vi "main_representacion.vi"(10 "Datos Leídos TyP":string[](array[string]), 11 "Datos Leídos Luz":string[](array[string])) -> ()   [LabVIEW 2021]
uses:
  Global 1.vi
panel:
  in  "Boolean 2":bool
  in  "Tab Control":T1(tab)
  out "Curvas luz y temperatura":cluster{"Ramp Pattern":dbl[], dbl[]}[](graph)
  in  "Load":bool
  in  "Export":bool
  in  "Curva de Luz":path
  in  "Curva de Temperatura":path
  in  "Ruta Luz":path
  in  "Ruta Temperatura":path
  in  "Integrate":bool
  in  "X1 (s)":dbl
  in  "X2 (s)":dbl
  out "Resultado":dbl
  in  "Load 2":bool
  in  "Load 3":bool
  out "Curvas  Luz":cluster{"Ramp Pattern":dbl[], u32[]}[](graph)
  in  "Luz 4":path
  in  "Luz 3":path
  in  "Luz 2":path
  in  "Luz 1":path
  in  "Temperatura 4":path
  in  "Temperatura 3":path
  in  "Temperatura 2":path
  in  "Temperatura 1":path
  out "Curvas Temperatura":cluster{"Ramp Pattern":dbl[], u32[]}[](graph)
  # "Glow Curves\nAnalysis"
  # "Área de integración"
  # "Curvas de Temperatura"
  # "Curvas de Luz"
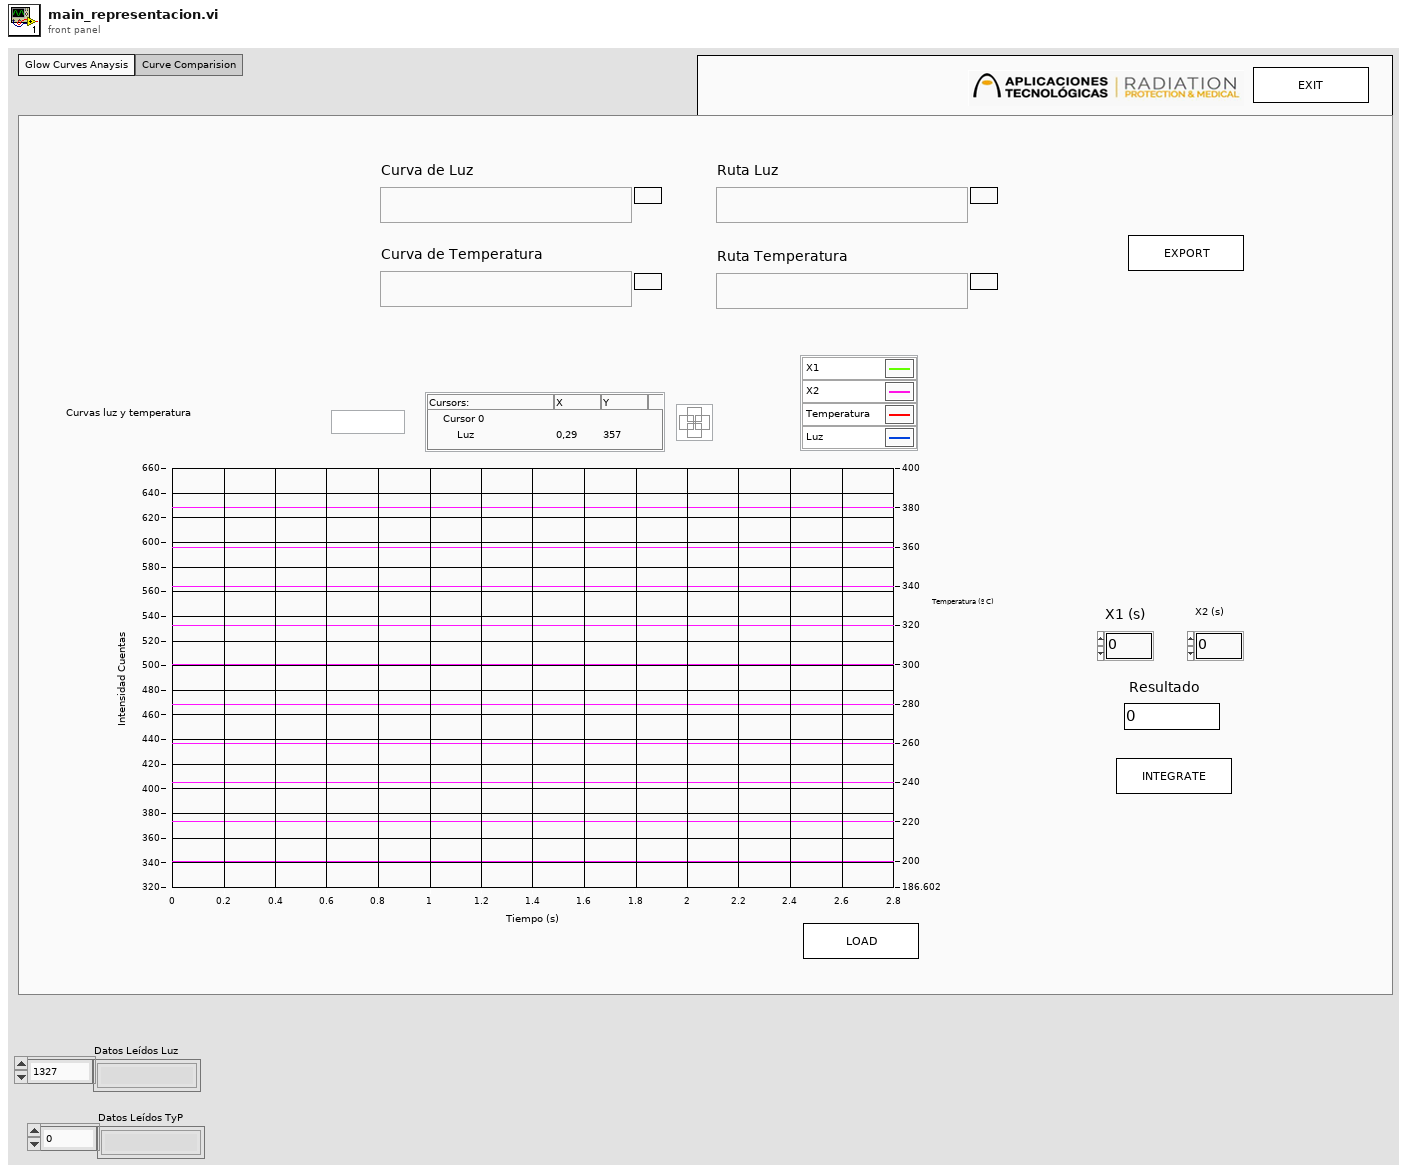
[diagram p1: front panel]
types:
  T1 = enum32{"Glow Curves Anaysis", "Curve Comparision"}
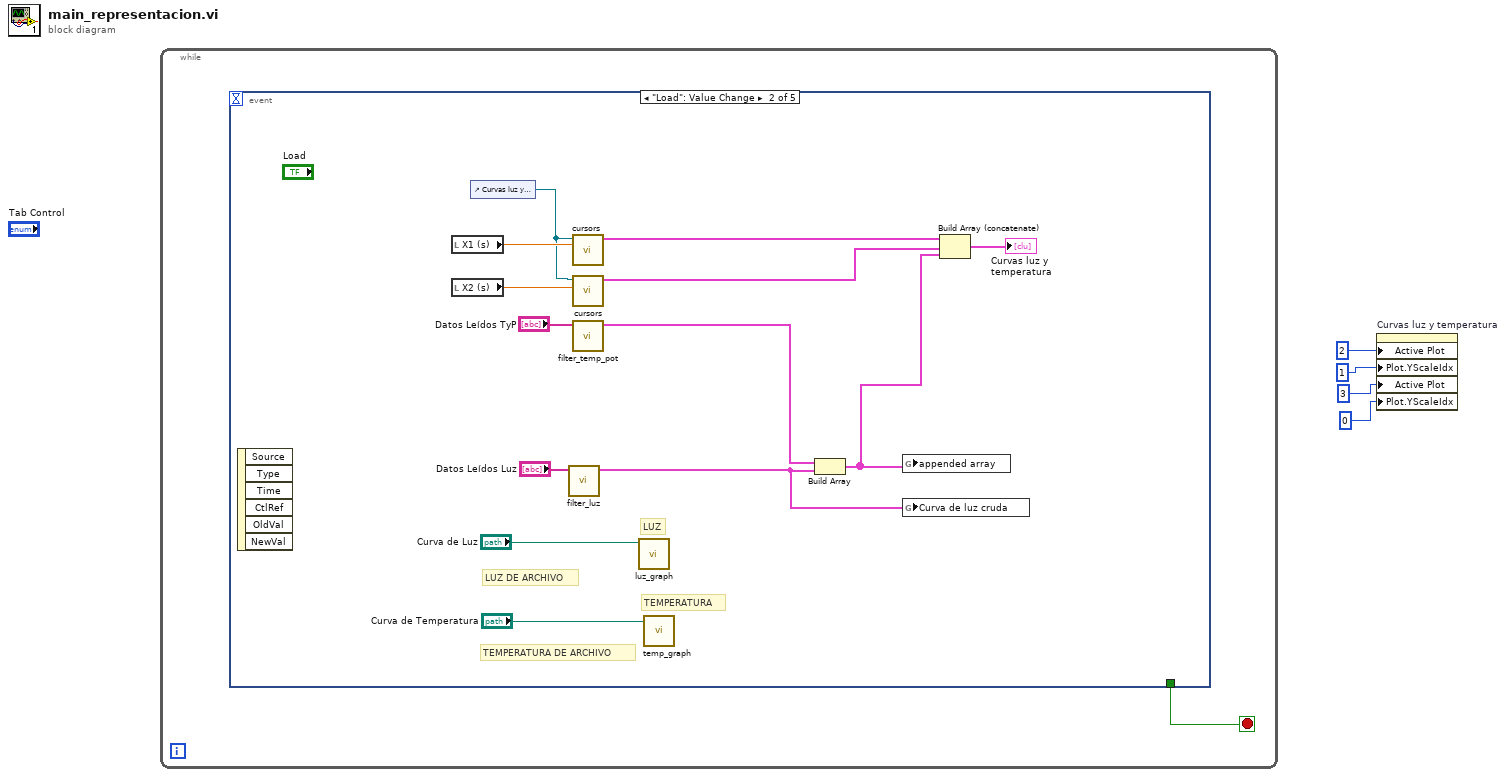
[diagram p0: block diagram]
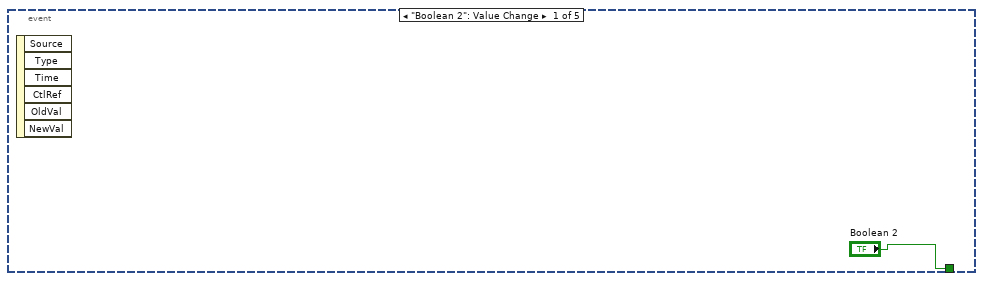
[diagram p2: hidden frame]
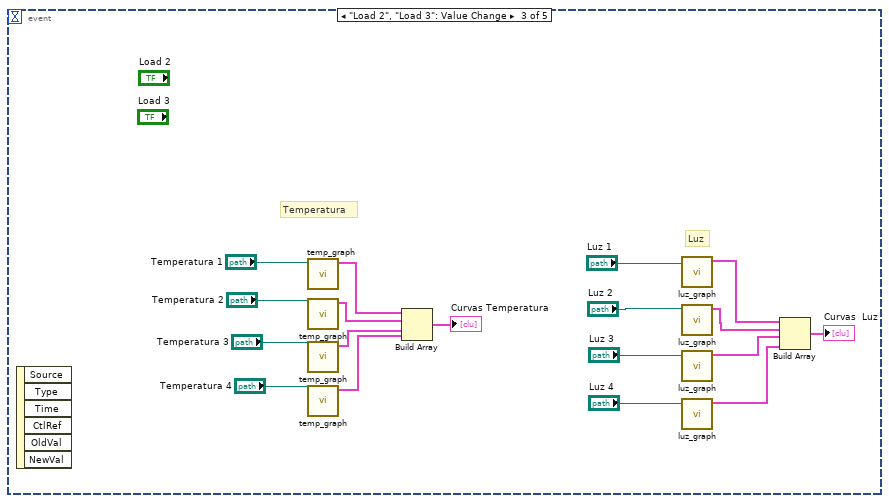
[diagram p3: hidden frame]
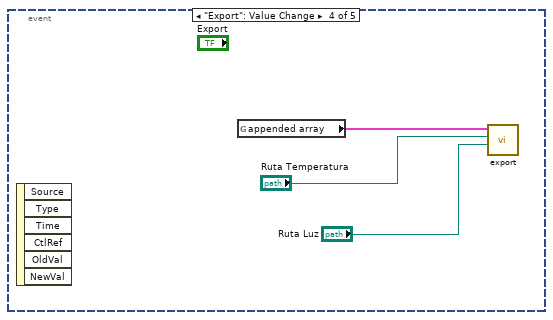
[diagram p4: hidden frame]
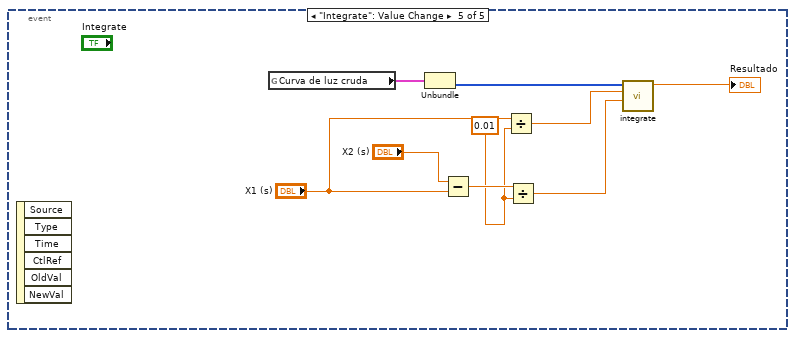
[diagram p5: hidden frame]
diagram:
  n1 = while {
    stop <- w5 stop-if-true
    n2 = event shown="[1] \"Load\": Value Change" {
      selector: _ -> [_ _ _ _ _]
      dyn-events: _ -> [_ _ _ _ _]
      timeout: _ -> [_ _ _ _ _]
      tunnel: ["Boolean 2" _ _ _ _] -> w5
      event "Boolean 2": Value Change {
        n3 = event-data() -> ()  [unwired: 1 in, 6 out]
      }
      event "Load": Value Change {
        # "TEMPERATURA"
        # "LUZ DE ARCHIVO"
        # "LUZ"
        # "TEMPERATURA DE ARCHIVO"
        n4 = event-data() -> ()  [unwired: 1 in, 6 out]
        n5 = local read "X1 (s)"() -> (w17:dbl)
        n6 = local read "X2 (s)"() -> (w15:dbl)
        n7 = control-ref of="Curvas luz y temperatura"() -> (w16:refnum<vi>)
        n8 = call "filter_luz.vi"("Datos Leídos Luz 3"="Datos Leídos Luz") -> ("Curva de luz"=w7:cluster{"Ramp Pattern":dbl[], u32[]})  [unwired: 10 in]
        n9 = call "cursors.vi"("X1 (s)"=w17, "XYGraph in"=w16) -> ("Cluster"=w14:cluster{dbl[], dbl[]})  [unwired: 9 in]
        n10 = call "cursors.vi"("X1 (s)"=w15, "XYGraph in"=w16) -> ("Cluster"=w13:cluster{dbl[], dbl[]})  [unwired: 9 in]
        n11 = call "filter_temp_pot.vi"("Datos Leídos T y P 2"="Datos Leídos TyP") -> ("Curva de temperatura"=w9:cluster{"Ramp Pattern":dbl[], u32[]})  [unwired: 9 in, 1 out]
        n12 = call "luz_graph.vi"("file path (dialog if empty)"="Curva de Luz") -> ()  [unwired: 10 in, 1 out]
        n13 = call "temp_graph.vi"("file path (dialog if empty) in"="Curva de Temperatura") -> ()  [unwired: 10 in, 1 out]
        n14 = Build Array(w9, w7) -> (w11:cluster{"Ramp Pattern":dbl[], u32[]}[])
        n15 = global write "Global 1.vi" "appended array"(w11) -> ()
        n16 = global write "Global 1.vi" "Curva de luz cruda"(w7) -> ()
        n17 = Build Array (concatenate)(w14, w13, w11) -> (→"Curvas luz y temperatura":cluster{"Ramp Pattern":dbl[], dbl[]}[])
      }
      event "Load 2", "Load 3": Value Change {
        # "Luz"
        # "Temperatura"
        n18 = event-data() -> ()  [unwired: 1 in, 6 out]
        n19 = call "temp_graph.vi"("file path (dialog if empty) in"="Temperatura 1") -> ("Curva de temperatura"=w29:cluster{"Ramp Pattern":dbl[], u32[]})  [unwired: 10 in]
        n20 = call "temp_graph.vi"("file path (dialog if empty) in"="Temperatura 2") -> ("Curva de temperatura"=w28:cluster{"Ramp Pattern":dbl[], u32[]})  [unwired: 10 in]
        n21 = call "temp_graph.vi"("file path (dialog if empty) in"="Temperatura 3") -> ("Curva de temperatura"=w27:cluster{"Ramp Pattern":dbl[], u32[]})  [unwired: 10 in]
        n22 = call "temp_graph.vi"("file path (dialog if empty) in"="Temperatura 4") -> ("Curva de temperatura"=w26:cluster{"Ramp Pattern":dbl[], u32[]})  [unwired: 10 in]
        n23 = Build Array(w29, w28, w27, w26) -> (→"Curvas Temperatura":cluster{"Ramp Pattern":dbl[], u32[]}[])
        n24 = call "luz_graph.vi"("file path (dialog if empty)"="Luz 1") -> ("Curva de luz"=w25:cluster{"Ramp Pattern":dbl[], u32[]})  [unwired: 10 in]
        n25 = call "luz_graph.vi"("file path (dialog if empty)"="Luz 2") -> ("Curva de luz"=w24:cluster{"Ramp Pattern":dbl[], u32[]})  [unwired: 10 in]
        n26 = call "luz_graph.vi"("file path (dialog if empty)"="Luz 3") -> ("Curva de luz"=w23:cluster{"Ramp Pattern":dbl[], u32[]})  [unwired: 10 in]
        n27 = call "luz_graph.vi"("file path (dialog if empty)"="Luz 4") -> ("Curva de luz"=w22:cluster{"Ramp Pattern":dbl[], u32[]})  [unwired: 10 in]
        n28 = Build Array(w25, w24, w23, w22) -> (→"Curvas  Luz":cluster{"Ramp Pattern":dbl[], u32[]}[])
      }
      event "Export": Value Change {
        n29 = event-data() -> ()  [unwired: 1 in, 6 out]
        n30 = global read "Global 1.vi" "appended array"() -> (w38:cluster{"Ramp Pattern":dbl[], u32[]}[])
        n31 = call "export.vi"("Ruta luz"="Ruta Luz", "Ruta Temp"="Ruta Temperatura", "Curva de Luz y Temperatura 3"=w38) -> ()  [unwired: 9 in]
      }
      event "Integrate": Value Change {
        w45 = 0.01 ("y")
        n32 = event-data() -> ()  [unwired: 1 in, 6 out]
        n33 = global read "Global 1.vi" "Curva de luz cruda"() -> (w49:cluster{"Ramp Pattern":dbl[], u32[]})
        n34 = Unbundle(w49) -> (w48:u32[])  [unwired: 1 out]
        n35 = Subtract(x="X2 (s)", y="X1 (s)") -> (x-y=w46:dbl)
        n36 = Divide(x="X1 (s)", y=w45) -> (x/y=w42:dbl)
        n37 = Divide(x=w46, y=w45) -> (x/y=w43:dbl)
        n38 = call "integrate.vi"("Longitud"=w43, "inicio"=w42, "Array"=w48) -> ("result"=→"Resultado":dbl)  [unwired: 8 in]
      }
    }
  }
  n39 = property on="Curvas luz y temperatura" class="XYGraph (strict)"("Active Plot"=u32 2, "Plot.YScaleIdx"=u32 1 ("Plot.Y Scale Index"), "Active Plot"=u32 3, "Plot.YScaleIdx"=u32 0 ("Plot.Y Scale Index")) -> ()  [unwired: 2 in, 2 out]
